vi "Data Storage - DRAM Support (B256).vi"(0 "data in":T2, 1 "input valid":bool, 3 "memory mode (F)":bool, 4 "priority (balanced)":T1, 5 "burst length (128)":u16=128, 6 "bypass DRAM FIFO (F)":bool, 7 "keep data (F)":bool, 8 "DRAM Memory":refnum<k21>, 9 "ready for output (T)":bool=TRUE, 10 "Memory Size":u32, 12 "DRAM Ready":bool, 13 "# of inputs available":u32, 14 "reset":bool, 15 "# of outputs ready for":u32) -> (19 "ready for input":bool, 20 "data out":T2, 21 "output valid":bool)   [LabVIEW 2018, in "Streaming FPGA.lvlib"]
doc: "DRAM Data Storage using the data type provided by the <B>Data Type (B256).ctl</B>. This storage can act as a FIFO (<B>memory mode</B> is false) or as a Memory (<B>memory mode</B> is true).\n\nWhen the DRAM Storage is used in Memory mode, it must be written first <B>Memory Size</B> number of times following a reset. No data output is returned during this write period. Once the Storage is written <B>Memory Size</B> number of times, the data output starts returning the data sequence stored in the memory, repeatedly. It is also possible to skip the DRAM Storage write period by setting the <B>keep data</B> input to true before applying the reset.\n\nThis VI uses the memory resource provided on the <B>DRAM Memory</B> input for storing the data elements. The <B>DRAM Memory</B> memory resource must use DRAM implementation and the data type must be the type provided by the <B>Data Type (B256).ctl</B> (array of 256 booleans). The <B>Memory Size</B> must be the requested number of elements parameter of the memory resource when the DRAM Storage is used in FIFO mode, or the number of elements the DRAM Storage should repeat when used in Memory mode. <B>DRAM Ready</B> must be set to true if the DRAM is ready. The <B>burst length</B> must be the DRAM read/write burst length the DRAM FIFO implementation should use (this must be less than the <B>Memory Size</B> and must be less than 1024). Use the <B>priority</B> input to select which operations to favor in FIFO mode: the \"favor writes\" option gives priority to DRAM writes, the \"favor reads\" option gives priority to DRAM reads, the \"balanced\" option balances between DRAM reads and writes. Set the <B>bypass DRAM FIFO</B> input to true to disable the use of the DRAM in FIFO mode.\n\n<B># of inputs available</B> must be the number of elements the upstream node can provide without blocking starting from the current cycle.\n<B># of outputs ready for</B> must be the number of elements the downstream node can accept without blocking starting from the current cycle.\n\nThe DRAM FIFO can hold at least <B>Memory Size</B> B256 elements."
uses:
  Streaming FPGA.lvlib
  Data Type (B256).ctl
  Data Storage - DRAM FIFO Priority.ctl
  <vilib>/rvi/DataTransferAndStorage/Container/Common/niFpgaContainerExecOnDevCompGetState.vi
  <vilib>/rvi/DataTransferAndStorage/Container/Common/niFpgaContainerGetUniqueNameForEmu.vi
  <vilib>/rvi/Memory/Memory_Emulation/niFpgaMemoryEmulationDramWriteAndRequestDataApplyByteEnables.vi
  <vilib>/rvi/Memory/Memory_Emulation/niFpgaMemoryEmulationCacheClearOnFirstRun.vi
  <vilib>/rvi/Memory/Memory_Emulation/nirvimemoryEmulationManagerCache_MakeExclusive.vi
  <vilib>/rvi/Memory/Memory_Emulation/nirvimemoryEmulationManagerCache_GetValue.vi
  <vilib>/rvi/Memory/Memory_Emulation/nirvimemoryEmulationManagerCache_InsertValue.vi
  <vilib>/Utility/error.llb/Clear Errors.vi
  <vilib>/rvi/Memory/Memory_Emulation/nirvimemoryEmulationManagerCache_ReleaseExclusive.vi
  <vilib>/rvi/Memory/Memory_Emulation/nirvimemoryEmulationManagerCache_SetValue.vi
  <vilib>/rvi/DataTransferAndStorage/Container/XNode/niFpgaContainer.xnode
  <vilib>/rvi/Memory/Memory_Emulation/niFpgaMemoryEmulationDramWriteAndRequestDataRefIn.vi
  <vilib>/rvi/Memory/Memory_Emulation/niFpgaMemoryEmulationDramRetrieveDataRefIn.vi
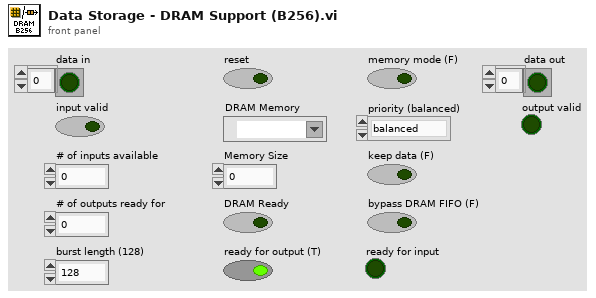
[diagram p1: front panel]
types:
  T1 = typedef "Streaming FPGA.lvlib/Data Storage - DRAM FIFO Priority.ctl" = enum16{"balanced", "favor writes", "favor reads"}
  T2 = typedef "Streaming FPGA.lvlib/Data Type (B256).ctl" = bool[]
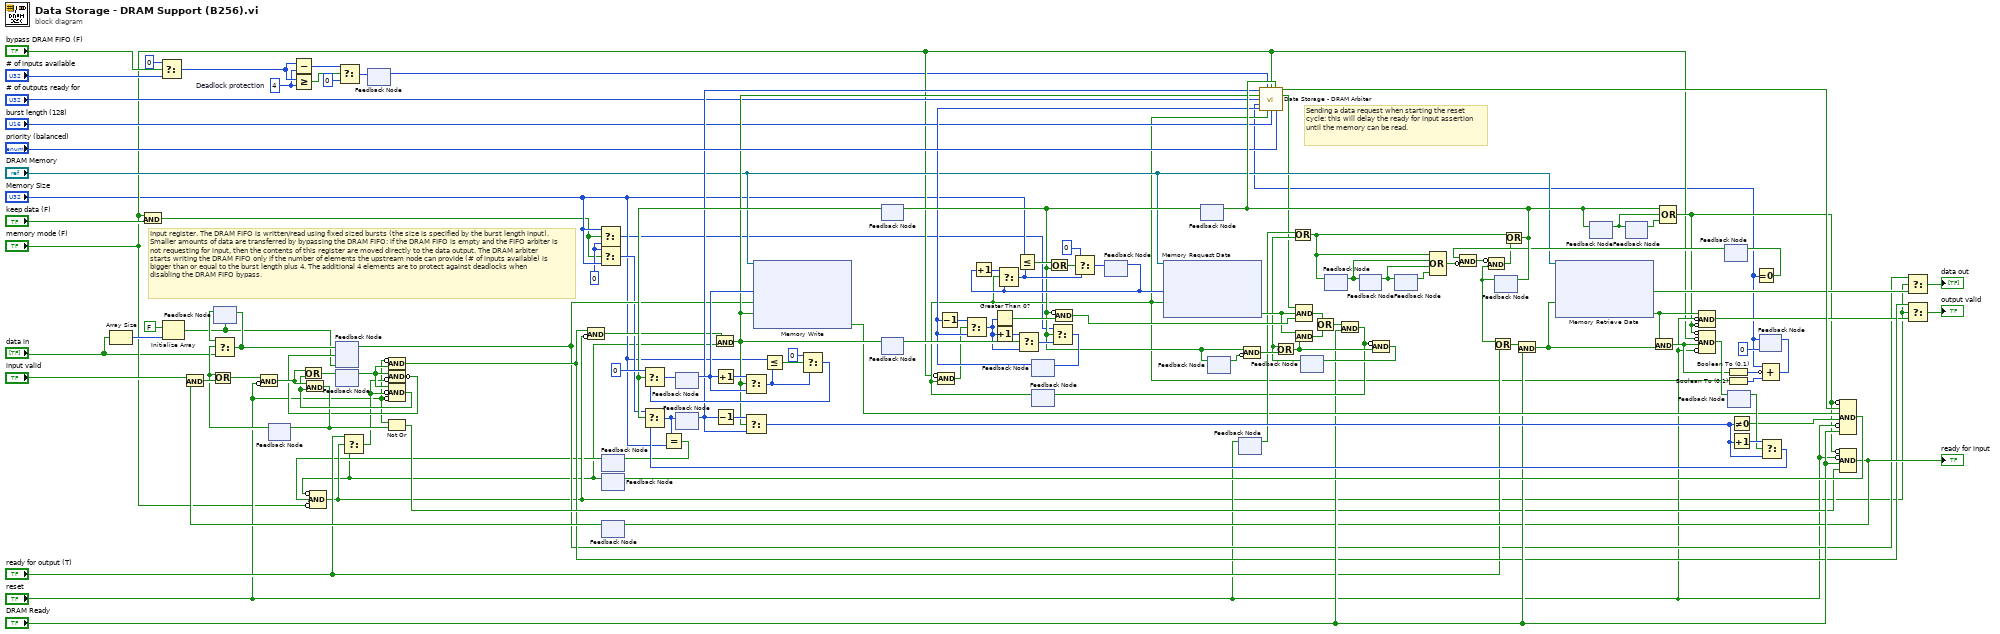
[diagram p0: block diagram]
diagram:
  w5 = u32 4  # Deadlock protection
  w20 = u32 0 ("t")
  # "Input register. The DRAM FIFO is written/read using fixed sized bursts (the size is specified by the burst length input). Smaller amounts of data are transferred by bypassing the DRAM FIFO: if the DRAM FIFO is empty and the FIFO arbiter is not requesting for input, then the contents of this register are moved directly to the data output. The DRAM arbiter starts writing the DRAM FIFO only if the number of elements the upstream node can provide (# of inputs available) is bigger than or equal to the burst length plus 4. The additional 4 elements are to protect against deadlocks when disabling the DRAM FIFO bypass."
  # "Sending a data request when starting the reset cycle: this will delay the ready for input assertion until the memory can be read."
  n1 = Array Size(array="data in") -> (size(s)=w128:i32)
  n2 = And(x="memory mode (F)", y="keep data (F)") -> (x .and. y?=w19:bool)
  n3 = Select(t=u32 0, s="bypass DRAM FIFO (F)", f="# of inputs available") -> (s? t:f=w6:u32)
  n4 = Initialize Array(FALSE, w128) -> (w12:bool[])
  n5 = feedback #1(w12) -> (w49:bool[])
  n6 = feedback #2() -> (w58:bool)  [unwired: 1 in]
  n7 = Select(t=w49, s=w58, f="data in") -> (s? t:f=w50:bool[])
  n8 = feedback-in #1(w50) -> ()
  n9 = Subtract(x=w6, y=w5) -> (x-y=w3:u32)
  n10 = Greater Or Equal?(x=w6, y=w5) -> (x >= y?=w4:bool)
  n11 = feedback #3(w12) -> (w33:bool[])
  n12 = feedback #4() -> (w52:bool)  [unwired: 1 in]
  n13 = Select(t=w3, s=w4, f=u32 0) -> (s? t:f=w1:u32)
  n14 = feedback-in #5(w1) -> ()
  n15 = feedback #5() -> (w7:u32)  [unwired: 1 in]
  n16 = Compound Arithmetic op=AND(invert "reset", w52) -> (w39:bool)
  n17 = Select(t="Memory Size", s=w19, f=w20) -> (s? t:f=w18:u32)
  n18 = Select(t=w20, s=w19, f="Memory Size") -> (s? t:f=w29:u32)
  n19 = feedback #6() -> (w9:bool)  [unwired: 1 in]
  n20 = feedback #7() -> (w8:bool)  [unwired: 1 in]
  n21 = Compound Arithmetic op=AND(invert w8, w9, invert "memory mode (F)") -> (w10:bool)
  n22 = Select(t="ready for output (T)", s=w10, f=w8) -> (s? t:f=w36:bool)
  n23 = Compound Arithmetic op=AND(w52, invert w36) -> (invert w51:bool)
  n24 = feedback-in #3(w50, w51) -> ()
  n25 = Compound Arithmetic op=AND(w52, invert w36, invert "reset") -> (w54:bool)
  n26 = Compound Arithmetic op=AND(w39, invert w10) -> (w34:bool)
  n27 = feedback #8() -> (w57:bool)  [unwired: 1 in]
  n28 = And(x="input valid", y=w57) -> (x .and. y?=w59:bool)
  n29 = Or(x=w58, y=w59) -> (x .or. y?=w56:bool)
  n30 = Compound Arithmetic op=AND(w56, invert "reset") -> (w55:bool)
  n31 = Or(x=w55, y=w54) -> (x .or. y?=w60:bool)
  n32 = And(x=w55, y=w54) -> (x .and. y?=w53:bool)
  n33 = feedback-in #2(w53) -> ()
  n34 = feedback-in #4(w60) -> ()
  n35 = Not Or(1:w53, 2:"reset") -> (0:w45:bool)
  n36 = feedback #9() -> (w103:u32)  [unwired: 1 in]
  n37 = feedback #10() -> (w81:u32)  [unwired: 1 in]
  n38 = And(x=w34, y=w8) -> (x .and. y?=w80:bool)
  n39 = Increment(x=w103) -> (x+1=w116:u32)
  n40 = Decrement(x=w81) -> (x-1=w114:u32)
  n41 = Select(t=w116, s=w80, f=w103) -> (s? t:f=w115:u32)
  n42 = Select(t=w114, s=w80, f=w81) -> (s? t:f=w90:u32)
  n43 = xnode ("Memory Write")("Address"=w103, "Data"=w33, "Input Valid"=w80, "Memory In"="DRAM Memory") -> ("Ready for Input"=w64:bool)  [unwired: 1 out]
  n44 = Less Or Equal?(x="Memory Size", y=w115) -> (x <= y?=w119:bool)
  n45 = Select(t=u32 0, s=w119, f=w115) -> (s? t:f=w102:u32)
  n46 = feedback #11() -> (w91:bool)  [unwired: 1 in]
  n47 = Select(t=u32 0, s=w91, f=w102) -> (s? t:f=w104:u32)
  n48 = feedback-in #9(w104) -> ()
  n49 = feedback-in #12(w80) -> ()
  n50 = feedback #12() -> (w117:bool)  [unwired: 1 in]
  n51 = feedback #13() -> (w77:u32)  [unwired: 1 in]
  n52 = Decrement(x=w77) -> (x-1=w123:u32)
  n53 = feedback #14() -> (w24:bool)  [unwired: 1 in]
  n54 = Compound Arithmetic op=AND(invert "memory mode (F)", w24) -> (w22:bool)
  n55 = Select(t=w123, s=w22, f=w77) -> (s? t:f=w93:u32)
  n56 = Greater Than 0?(x=w93) -> (x > 0?=w96:bool)
  n57 = Increment(x=w93) -> (x+1=w124:u32)
  n58 = Select(t=w124, s=w117, f=w93) -> (s? t:f=w97:u32)
  n59 = feedback #15() -> (w109:u32)  [unwired: 1 in]
  n60 = Increment(x=w109) -> (x+1=w121:u32)
  n61 = Select(t=w121, s=w24, f=w109) -> (s? t:f=w112:u32)
  n62 = Less Or Equal?(x="Memory Size", y=w112) -> (x <= y?=w111:bool)
  n63 = xnode ("Memory Request Data")("Address"=w109, "Input Valid"=w24, "Memory In"="DRAM Memory") -> ("Ready for Input"=w87:bool)  [unwired: 1 out]
  n64 = feedback #16() -> (w82:bool)  [unwired: 1 in]
  n65 = feedback-in #11(w82) -> ()
  n66 = Or(x=w111, y=w82) -> (x .or. y?=w110:bool)
  n67 = Select(t=w18, s=w82, f=w97) -> (s? t:f=w98:u32)
  n68 = feedback-in #13(w98) -> ()
  n69 = Compound Arithmetic op=AND(invert w82, w96) -> (w126:bool)
  n70 = Select(t=u32 0, s=w110, f=w112) -> (s? t:f=w113:u32)
  n71 = feedback-in #15(w113) -> ()
  n72 = feedback-in #17(w82) -> ()
  n73 = feedback #17() -> (w89:bool)  [unwired: 1 in]
  n74 = feedback #18() -> (w74:bool)  [unwired: 1 in]
  n75 = feedback-in #18("reset") -> ()
  n76 = Compound Arithmetic op=AND(w82, invert w89) -> (w88:bool)
  n77 = feedback #19() -> (w71:bool)  [unwired: 1 in]
  n78 = Or(x=w71, y=w88) -> (x .or. y?=w84:bool)
  n79 = Or(x=w74, y=w71) -> (x .or. y?=w17:bool)
  n80 = And(x=w87, y=w84) -> (x .and. y?=w85:bool)
  n81 = feedback-in #20(w17) -> ()
  n82 = feedback #20() -> (w16:bool)  [unwired: 1 in]
  n83 = feedback #21() -> (w15:bool)  [unwired: 1 in]
  n84 = feedback-in #21(w16) -> ()
  n85 = feedback #22() -> (w70:bool)  [unwired: 1 in]
  n86 = feedback-in #22(w15) -> ()
  n87 = Compound Arithmetic op=OR(w17, w16, w15, w70) -> (w69:bool)
  n88 = feedback #23() -> (w66:bool)  [unwired: 1 in]
  n89 = Or(x=w66, y="ready for output (T)") -> (x .or. y?=w106:bool)
  n90 = And(x=w106, y="DRAM Ready") -> (x .and. y?=w61:bool)
  n91 = xnode ("Memory Retrieve Data")("Ready for Output"=w61, "Memory In"="DRAM Memory") -> ("Data"=w41:bool[], "Output Valid"=w95:bool)  [unwired: 1 out]
  n92 = feedback #24() -> (w73:bool)  [unwired: 1 in]
  n93 = feedback #25() -> (w72:bool)  [unwired: 1 in]
  n94 = feedback-in #25(w73) -> ()
  n95 = And(x=w95, y=w61) -> (x .and. y?=w92:bool)
  n96 = feedback #26() -> (w130:bool)  [unwired: 1 in]
  n97 = Compound Arithmetic op=AND(w130, invert w69) -> (w67:bool)
  n98 = Compound Arithmetic op=AND(invert w67, w66) -> (w68:bool)
  n99 = Or(x=w17, y=w68) -> (x .or. y?=w131:bool)
  n100 = feedback-in #16(w131) -> ()
  n101 = feedback-in #23(w131) -> ()
  n102 = feedback-in #24(w131) -> ()
  n103 = Compound Arithmetic op=OR(w131, w73, w72) -> (w28:bool)
  n104 = Compound Arithmetic op=AND(w95, invert "reset", invert w28) -> (w38:bool)
  n105 = Compound Arithmetic op=AND(invert w28, invert "memory mode (F)", w92, invert "reset") -> (w100:bool)
  n106 = Boolean To (0,1)(Boolean=w92) -> (0, 1=w108:i16)
  n107 = Boolean To (0,1)(Boolean=w24) -> (0, 1=w107:i16)
  n108 = feedback #27() -> (w99:bool)  [unwired: 1 in]
  n109 = feedback-in #27(w100) -> ()
  n110 = Not Equal To 0?(x=w90) -> (x != 0?=w94:bool)
  n111 = Increment(x=w90) -> (x+1=w120:u32)
  n112 = feedback #28(i16 0 ("t")) -> (w11:i16)
  n113 = call "Data Storage - DRAM Arbiter.vi"("# of empty slots available"=w81, "# of inputs available"=w7, "memory mode"="memory mode (F)", "reset"=w131, "input write"=w80, "# of outputs ready for"="# of outputs ready for", "# of pending reads"=w11, "# of words available"=w77, "request for data"=w24, "burst length"="burst length (128)", "priority (balanced)"="priority (balanced)") -> ("write enable"=w79:bool, "read enable"=w32:bool)  [unwired: 3 in]
  n114 = Compound Arithmetic op=AND(w32, w87, w126) -> (w86:bool)
  n115 = Or(x=w86, y=w85) -> (x .or. y?=w63:bool)
  n116 = And(x=w63, y="DRAM Ready") -> (x .and. y?=w62:bool)
  n117 = feedback-in #14(w62) -> ()
  n118 = Compound Arithmetic op=AND(invert w62, w84) -> (w83:bool)
  n119 = feedback-in #19(w83) -> ()
  n120 = Equal To 0?(x=w11) -> (x = 0?=w129:bool)
  n121 = feedback-in #26(w129) -> ()
  n122 = Select(t=w120, s=w99, f=w90) -> (s? t:f=w101:u32)
  n123 = Select(t=w29, s=w91, f=w101) -> (s? t:f=w43:u32)
  n124 = Equal?(x=w43, y="Memory Size") -> (x = y?=w42:bool)
  n125 = feedback-in #6(w42) -> ()
  n126 = feedback-in #10(w43) -> ()
  n127 = Compound Arithmetic op=ADD(w11, invert w108, w107) -> (w65:i16)
  n128 = feedback-in #28(w65) -> ()
  n129 = Compound Arithmetic op=AND(invert w28, w79, w64, w94, invert "reset", "DRAM Ready") -> (w47:bool)
  n130 = feedback-in #7(w47) -> ()
  n131 = Compound Arithmetic op=AND(invert w28, invert "reset", "DRAM Ready", w45) -> (w44:bool)
  "ready for input" <- w44
  n132 = feedback-in #8(w44) -> ()
  n133 = Select(t=w33, s=w10, f=w41) -> (s? t:f=→"data out":bool[])
  n134 = Select(t=w39, s=w10, f=w38) -> (s? t:f=→"output valid":bool)
